vi "Fetch Raw Unit Data.vi"(0 "VISA resource name":refnum<visa-resource-name>, 5 "Start Channel (1)":string="0001", 7 "End Channel (1)":string="0001", 11 "error in (no error)":errorcluster) -> (4 "VISA resource name out":refnum<visa-resource-name>, 8 "Unit Data":string, 15 "error out":errorcluster)   [LabVIEW 2020, in "Yokogawa GX Series.lvlib"]
doc: "This VI gets the decimal place and units by ASCII."
uses:
  <instrlib>/Yokogawa GX Series/Yokogawa GX Series.lvlib
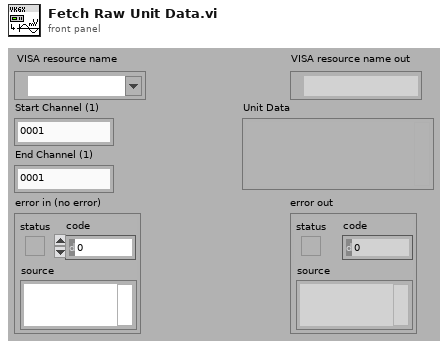
[diagram p1: front panel]
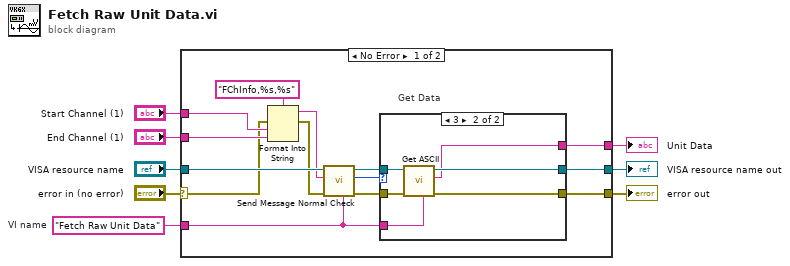
[diagram p0: block diagram]
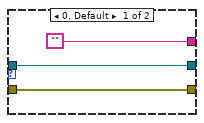
[diagram p2: hidden frame]
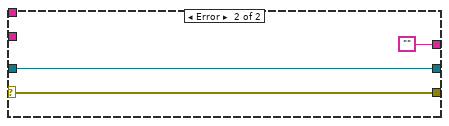
[diagram p3: hidden frame]
diagram:
  w4 = "Fetch Raw Unit Data"  # VI name
  n1 = case shown="No Error" "error in (no error)" {
    selector: "error in (no error)" -> [w9 w33]
    tunnel: [w22 w34] -> w8
    tunnel: [w21 w33] -> w7
    tunnel: [w20 ""] -> w6
    tunnel: "VISA resource name" -> [w18 w34]
    tunnel: w4 -> [w15 _]
    tunnel: "Start Channel (1)" -> [w14 _]
    tunnel: "End Channel (1)" -> [w13 _]
    frame No Error {
      # "Get Data"
      n2 = Format Into String(format string="FChInfo,%s,%s", error in=w9, w14, w13) -> (resulting string=w17:string, error out=w16:errorcluster)  [unwired: 1 in]
      n3 = call <instrlib>:"Send Message Normal Check.vi"("Source (\"\")"=w15, "error in (no error)"=w16, "Send Message (\"\")"=w17, "VISA resource name"=w18) -> ("error out"=w12:errorcluster, "Response Type"=w10:i32, "VISA resource name out"=w11:refnum<visa-resource-name>)  [unwired: 1 in, 4 out]
      n4 = case shown="3" w10 {
        tunnel: ["" w27] -> w20
        tunnel: [w24 w26] -> w21
        tunnel: [w25 w29] -> w22
        tunnel: w11 -> [w25 w31]
        tunnel: w12 -> [w24 w30]
        tunnel: w15 -> [_ w28]
        frame 0, Default {
        }
        frame 3 {
          n5 = call <instrlib>:"Get ASCII.vi"("Source (\"\")"=w28, "error in (no error)"=w30, "VISA resource name"=w31) -> ("error out"=w26:errorcluster, "ASCII Data"=w27:string, "VISA resource name out"=w29:refnum<visa-resource-name>)  [unwired: 6 out]
        }
      }
    }
    frame Error {
    }
  }
  "error out" <- w7
  "VISA resource name out" <- w8
  "Unit Data" <- w6
